vi "NI VeriStand - Print Debug String.vi"(7 "Attribute":T1=7 items=["Plain White"=7, "Bold White"=15, "Bold Blue"=9, "Bold Green"=10, "Bold Red"=12], 8 "error in (no error)":errorcluster, 10 "Add to log file? (F)":bool, 11 "Message":string) -> (0 "error out":errorcluster)   [LabVIEW 2020, in "Custom Device Utility Library.lvlib"]
doc: "Prints a string to the console and if desired, to the NI VeriStand data log. This VI only operates within the context of the NI VeriStand engine."
uses:
  <vilib>/NI VeriStand/Custom Device Tools/Custom Device Utility Library/Custom Device Utility Library.lvlib
  <vilib>/NI VeriStand/Custom Device Tools/Custom Device Utility Library/RT Debug String Color Spec.ctl
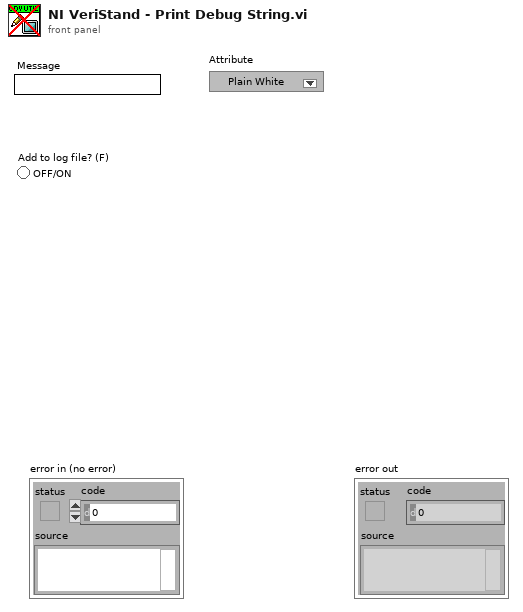
[diagram p1: front panel]
types:
  T1 = typedef "Custom Device Utility Library.lvlib/RT Debug String Color Spec.ctl" = u16
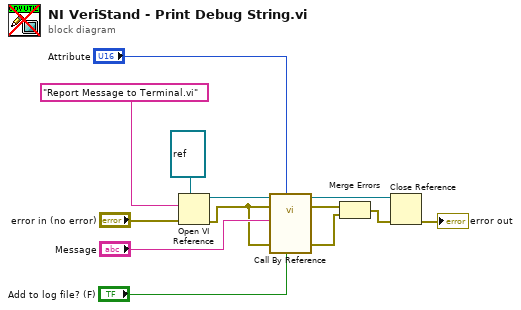
[diagram p0: block diagram]
diagram:
  n1 = Open VI Reference(type specifier VI Refnum (for type only)=refnum<vi> refnum, vi path="Report Message to Terminal.vi", error in (no error)="error in (no error)") -> (vi reference=w10:refnum<vi>, error out=w8:errorcluster)  [unwired: 3 out]
  n2 = call-by-ref "?"(reference=w10, error in=w8, "Add to log file? (T)"="Add to log file? (F)", "Color (Plain White)"="Attribute", 8:"error in (no error)"=w8, "Message"="Message") -> (reference out=w3:refnum<vi>, error out=w7:errorcluster, 0:"error out"=w6:errorcluster)  [unwired: 7 in]
  n3 = Merge Errors(w7, w6) -> (w2:errorcluster)
  n4 = Close Reference(reference=w3, error in (no error)=w2) -> (error out=→"error out":errorcluster)
